vi "Update AO DC.vi"(8 "error in (no error)":errorcluster, 10 "AO.DC (V)":dbl[](array[numeric]), 11 "Generator in":refnum<class "Generator.lvclass">) -> (0 "error out":errorcluster, 3 "Generator out":refnum<class "Generator.lvclass">)   [LabVIEW 2019, in "Generator.lvclass"]
uses:
  Generator.lvclass
  Generator.lvclass/Generator.ctl
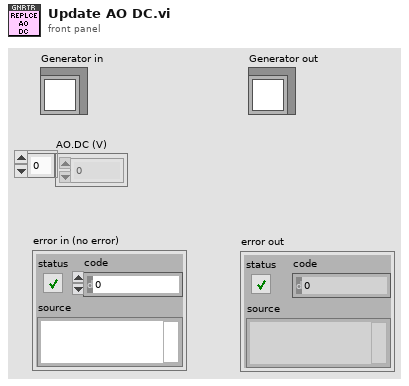
[diagram p1: front panel]
types:
  T1 = typedef "Generator.lvclass/AO.Channel--Cluster--Array.ctl" = T2[]
  T2 = typedef "Generator.lvclass/AO.Channel--Cluster.ctl" = cluster{"Enable?":bool, "Channel":i32, "Amplitude":dbl, "Offset":dbl, "Frequency":dbl, "Phase":dbl, "Function":T3, "Sweeping?":bool, "Limit AC?":bool, "Limit DC?":bool, "Duty Cycle?":bool, "Duty Cycle":dbl}
  T3 = typedef "Generator.lvclass/AO.Channel.Function--Enum.ctl" = enum16{"sine", "square", "triangle", "saw"}
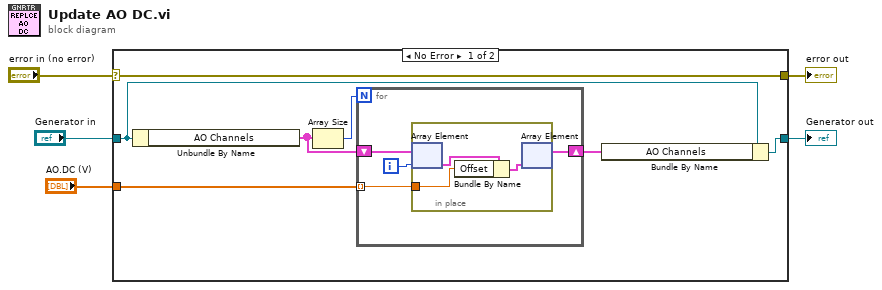
[diagram p0: block diagram]
diagram:
  n1 = case shown="No Error" "error in (no error)" {
    selector: "error in (no error)" -> [w9 w21]
    tunnel: "AO.DC (V)" -> [w12 _]
    tunnel: "Generator in" -> [w11 w20]
    tunnel: [w10 w20] -> w2
    tunnel: [w9 w21] -> w1
    frame No Error {
      n2 = Unbundle By Name(w11) -> ("AO Channels"=w8:T1)
      n3 = Array Size(array=w8) -> (size(s)=w7:i32)
      n4 = for {
        N: w7 -> [_]
        tunnel: w12 -> [w16] mode=indexing
        shift-right: [w14] -> w6
        shift-left: w8 -> [w15]
        i -> [w13]
        n5 = in-place {
          in-place-border: w16 -> [w19]
          n6 = in-place-array #1(w15, w13) -> (w18:T2)
          n7 = Bundle By Name(cluster=w18, "Offset"=w19) -> (w17:T2)
          n8 = in-place-array #1(w17) -> (w14:T1)  [unwired: 1 out]
        }
      }
      n9 = Bundle By Name(cluster=w11, "AO Channels"=w6) -> (w10:refnum<class "Generator.lvclass">)
    }
    frame Error {
    }
  }
  "Generator out" <- w2
  "error out" <- w1
